vi "SLSC Set Reservation Values.vi"(8 "error in (no error)":errorcluster, 9 "Reservation Access":i32(ring)=3 items=["None"=0, "Read Only"=1, "Read/Write"=3], 10 "Reservation Group":string, 11 "Section Ref in":T1 format="%.0x") -> (0 "error out":errorcluster, 3 "Item Ref out":T1 format="%.0x")   [LabVIEW 2020, in "SLSC EDS System Explorer.lvlib"]
uses:
  System Explorer/SLSC EDS System Explorer.lvlib
  <vilib>/NI VeriStand/Custom Device API/Custom Device Item Ref.ctl
  Shared/Constants.vi
  <vilib>/NI VeriStand/Custom Device API/Set Item Property (String).vi
  <vilib>/NI VeriStand/Custom Device API/Set Item Property (I32).vi
  Shared/SLSC EDS Shared.lvlib
  <vilib>/NI VeriStand/Custom Device API/Custom Device API.lvlib
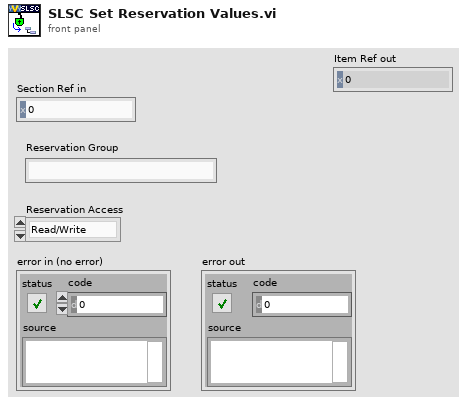
[diagram p1: front panel]
types:
  T1 = typedef "Custom Device API.lvlib/Custom Device Item Ref.ctl" = u64
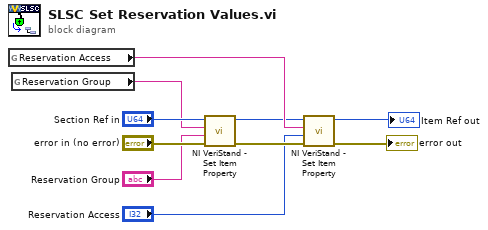
[diagram p0: block diagram]
diagram:
  n1 = global read "Constants.vi" "Reservation Access"() -> (w6:string)
  n2 = global read "Constants.vi" "Reservation Group"() -> (w4:string)
  n3 = call-poly <vilib>:"NI VeriStand - Set Item Property.vi"("error in (no error)"="error in (no error)", "Value"="Reservation Group", "Property Name"=w4, "Item Ref in"="Section Ref in") -> ("error out"=w9:errorcluster, "Item Ref out"=w5:T1)  [unwired: 5 in, 1 out]
  n4 = call-poly <vilib>:"NI VeriStand - Set Item Property.vi"("error in (no error)"=w9, "Value"="Reservation Access", "Property Name"=w6, "Item Ref in"=w5) -> ("error out"=→"error out":errorcluster, "Item Ref out"=→"Item Ref out":T1)  [unwired: 5 in, 1 out]
